vi "ex8_traffic light.vi"() -> ()   [LabVIEW 2018]
panel:
  in  "Boolean 5":bool
  out "Boolean 4":bool
  out "Numeric":dbl
  in  "stop":bool
  out "Boolean 3":bool
  out "Boolean 2":bool
  out "Boolean":bool
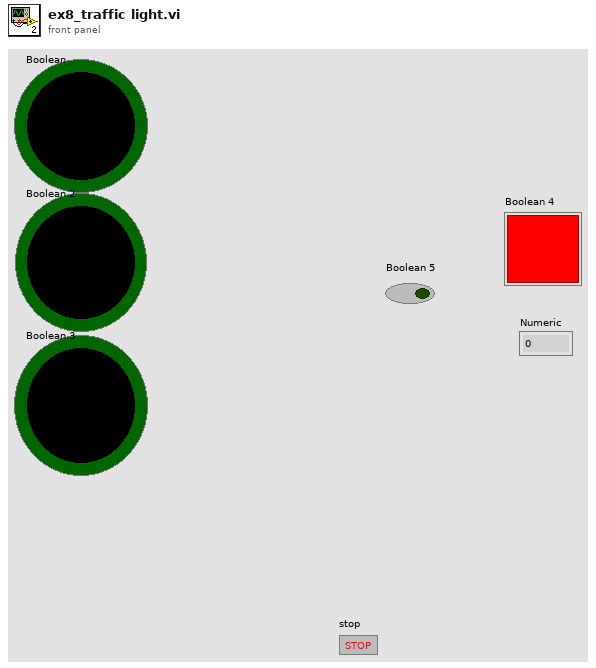
[diagram p1: front panel]
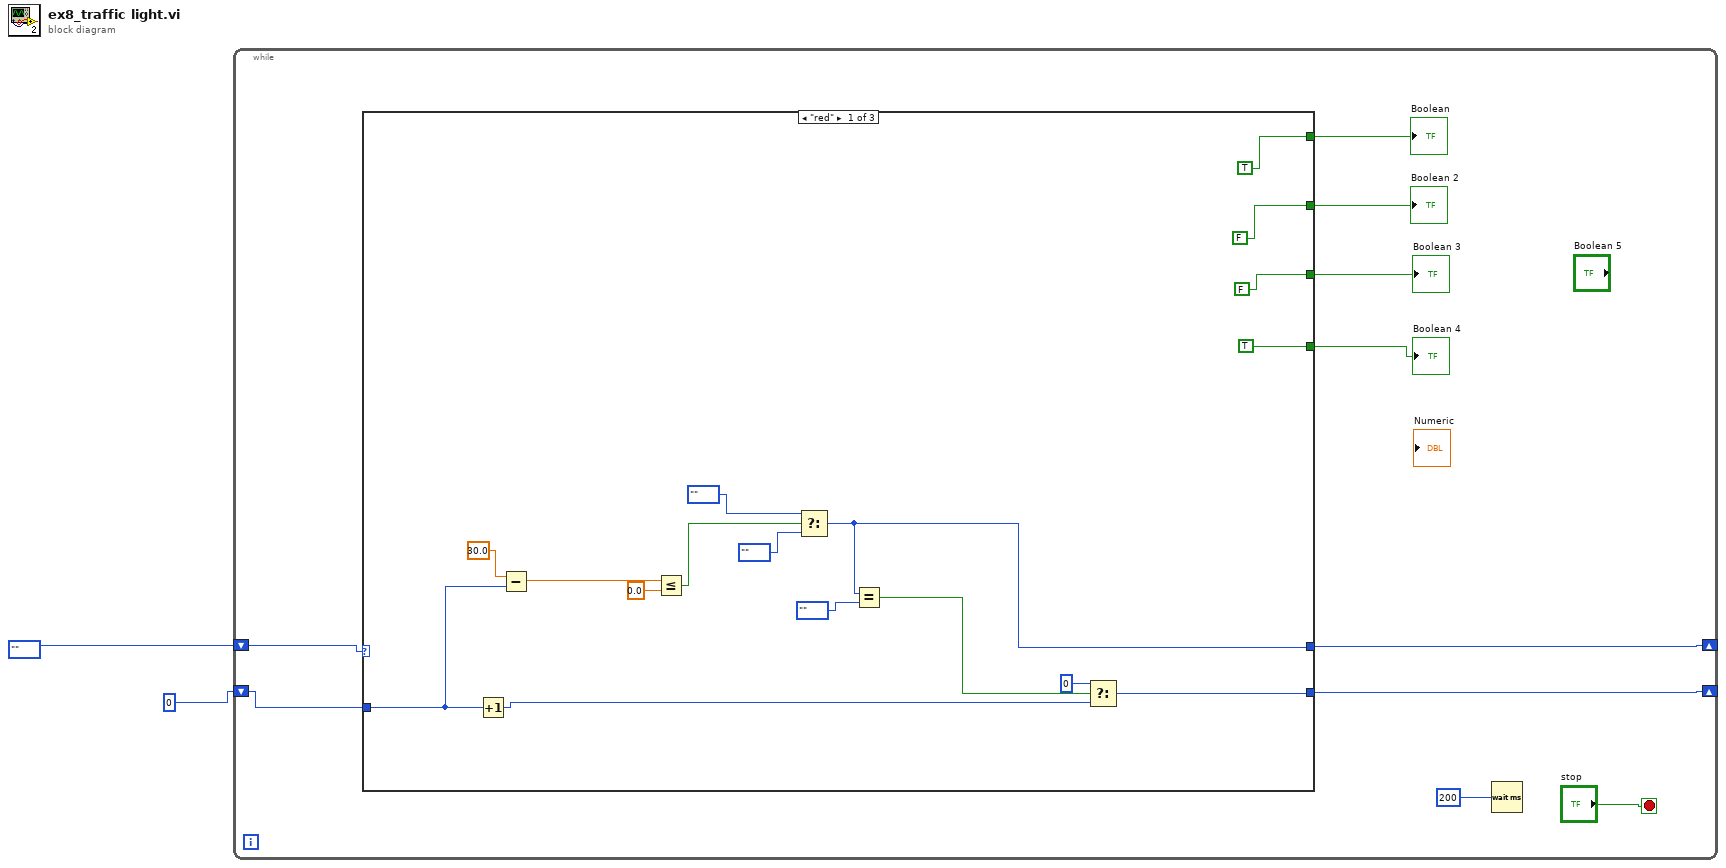
[diagram p0: block diagram]
diagram:
  n1 = while {
    shift-right: [w7] -> _
    shift-left: enum16{""}."" -> [w11]
    shift-right: [w8] -> _
    shift-left: 0 -> [w9]
    stop <- "stop" stop-if-true
    n2 = case shown="\"red\"" w11 {
      tunnel: w9 -> [w26 _ _]
      tunnel: [w18 _ _] -> w8
      tunnel: [w17 _ _] -> w7
      tunnel: [TRUE _ _] -> w6
      tunnel: [FALSE _ _] -> w5
      tunnel: [FALSE _ _] -> w4
      tunnel: [TRUE _ _] -> w3
      frame 1 {
        n3 = Increment(x=w26) -> (x+1=w25:i32)
        n4 = Subtract(x=30.0, y=w26) -> (x-y=w28:dbl)
        n5 = Less Or Equal?(x=w28, y=0.0) -> (x <= y?=w21:bool)
        n6 = Select(t=enum16{""}."", s=w21, f=enum16{""}."") -> (s? t:f=w17:enum16{""})
        n7 = Equal?(x=w17, y=enum16{""}."") -> (x = y?=w20:bool)
        n8 = Select(t=0, s=w20, f=w25) -> (s? t:f=w18:i32)
      }
      frame 2 {
      }
      frame "" {
      }
    }
    "Boolean 3" <- w4
    "Boolean 2" <- w5
    "Boolean" <- w6
    "Boolean 4" <- w3
    n9 = Wait (ms)(milliseconds to wait=u32 200 ("millisecond timer value")) -> ()  [unwired: 1 out]
  }
